vi "S4GUI.vi"(7 "Tab ObsEng":enum32{"Obs", "CCD modes", "Eng"}(tab)) -> ()   [LabVIEW 2018] (continued)
            w9668 = i16 1 items=["Cooler OFF", "Cooler ON"] ("Cooler ON/OFF")
          }
        }
        n4075 = Concatenate Strings("SET COOLER " ("User Event"), w9632, "CLICKED - CH4" ("User Event")) -> (w9636:string)
        n4076 = call-dynamic "Write User Event.vi"("error in (no error)"=w9633, "User Event"=w9636, "S4GUI in"=w9634) -> ("error out"=w9630:errorcluster, "S4GUI out"=w9631:refnum<class "S4GUI.lvclass">)  [unwired: 7 in]
        n4077 = call-dynamic "Read AcquisitionD.vi"("error in (no error)"=w9630, "S4ACS_GUI in"=w9631) -> ("error out"=w9640:errorcluster, "Acquisition.lvclass"=w9643:refnum<class "Acquisition.lvclass">, "S4ACS_GUI out"=w9644:refnum<class "S4GUI.lvclass">)  [unwired: 7 in]
        n4078 = call-dynamic "Read Channel.vi"("error in (no error)"=w9640, "Acquisition in"=w9643) -> ("error out"=w9649:errorcluster, "Channel.lvclass"=w9654:refnum<class "Channel.lvclass">, "Acquisition out"=w9657:refnum<class "Acquisition.lvclass">)  [unwired: 7 in]
        n4079 = call-dynamic "Read Interface.vi"("error in (no error)"=w9649, "Channel in"=w9654) -> ("error out"=w9648:errorcluster, "Interface.lvclass"=w9651:refnum<class "Interface.lvclass">, "Channel out"=w9653:refnum<class "Channel.lvclass">)  [unwired: 7 in]
        n4080 = call-dynamic "Write Cooler ON_OFF.vi"("error in (no error)"=w9648, "Cooler ON/OFF"=w9646, "Interface in"=w9651) -> ("error out"=w9647:errorcluster, "Interface out"=w9650:refnum<class "Interface.lvclass">)  [unwired: 7 in]
        n4081 = call-dynamic "Write Interface.vi"("error in (no error)"=w9647, "Interface.lvclass"=w9650, "Channel in"=w9653) -> ("error out"=w9639:errorcluster, "Channel out"=w9652:refnum<class "Channel.lvclass">)  [unwired: 7 in]
        n4082 = call-dynamic "Read State Machine.vi"("error in (no error)"=w9639, "Device in"=w9652) -> ("error out"=w9661:errorcluster, "State Machine.lvclass"=w9662:refnum<class "State Machine.lvclass">, "Device out"=w9658:refnum<class "Channel.lvclass">)  [unwired: 7 in]
        n4083 = call "Next State.vi"("error in (no error)"=w9661, "New_State"=u32 30, "State Machine in"=w9662) -> ("error out"=w9656:errorcluster, "State Machine out"=w9659:refnum<class "State Machine.lvclass">)  [unwired: 7 in]
        n4084 = call-dynamic "Write State Machine.vi"("error in (no error)"=w9656, "State Machine.lvclass"=w9659, "Device in"=w9658) -> ("error out"=w9655:errorcluster, "Device out"=w9645:refnum<class "Channel.lvclass">)  [unwired: 7 in]
        n4085 = call-dynamic "Write Channel.vi"("error in (no error)"=w9655, "Channel.lvclass"=w9645, "Acquisition in"=w9657) -> ("error out"=w9641:errorcluster, "Acquisition out"=w9642:refnum<class "Acquisition.lvclass">)  [unwired: 7 in]
        n4086 = call-dynamic "Write AcquisitionD.vi"("error in (no error)"=w9641, "Acquisition.lvclass"=w9642, "S4ACS_GUI in"=w9644) -> ("error out"=w9663:errorcluster, "S4ACS_GUI out"=w9664:refnum<class "S4GUI.lvclass">)  [unwired: 7 in]
      }
      event "Set Temp 1": Value Change {
        n4087 = event-data() -> ("NewVal"=w9669:bool)  [unwired: 1 in]
        n4088 = case shown="True" w9669 {
          tunnel: w9673 -> [w9675 w9702]
          tunnel: w9672 -> [w9674 w9701]
          tunnel: [w9674 w9691] -> w9671
          tunnel: [w9675 w9692] -> w9670
          frame False {
          }
          frame True {
            # "Carrega a maior temperatura\nentre target atual e o target do controle."
            # "Carrega o valor da temperatura target de acordo com a conf CCD"
            n4089 = call-dynamic "Read AcquisitionA.vi"("error in (no error)"=w9701, "S4ACS_GUI in"=w9702) -> ("error out"=w9705:errorcluster, "Acquisition.lvclass"=w9704:refnum<class "Acquisition.lvclass">, "S4ACS_GUI out"=w9711:refnum<class "S4GUI.lvclass">)  [unwired: 7 in]
            n4090 = call-dynamic "Read Channel.vi"("error in (no error)"=w9705, "Acquisition in"=w9704) -> ("error out"=w9721:errorcluster, "Channel.lvclass"=w9720:refnum<class "Channel.lvclass">, "Acquisition out"=w9708:refnum<class "Acquisition.lvclass">)  [unwired: 7 in]
            n4091 = call-dynamic "ValidateConfig.vi"("error in (no error)"=w9721, "Channel in"=w9720) -> ("error out"=w9727:errorcluster, "Channel out"=w9726:refnum<class "Channel.lvclass">)  [unwired: 7 in, 1 out]
            n4092 = call-dynamic "Read Interface.vi"("error in (no error)"=w9727, "Channel in"=w9726) -> ("error out"=w9723:errorcluster, "Interface.lvclass"=w9722:refnum<class "Interface.lvclass">, "Channel out"=w9716:refnum<class "Channel.lvclass">)  [unwired: 7 in]
            n4093 = call-dynamic "Read Temperature.vi"("error in (no error)"=w9723, "Interface in"=w9722) -> ("error out"=w9724:errorcluster, "Temperature"=w9729:i8, "Interface out"=w9725:refnum<class "Interface.lvclass">)  [unwired: 7 in]
            n4094 = Greater?(x=w9729, y="Target Temp 1") -> (0:w9728:bool)
            n4095 = Select(t=w9729, s=w9728, f="Target Temp 1") -> (s? t:f=w9695:i8)
            n4096 = call-dynamic "Write Temperature.vi"("error in (no error)"=w9724, "Temperature"=w9695, "Interface in"=w9725) -> ("error out"=w9718:errorcluster, "Interface out"=w9715:refnum<class "Interface.lvclass">)  [unwired: 7 in]
            n4097 = call-dynamic "Write Interface.vi"("error in (no error)"=w9718, "Interface.lvclass"=w9715, "Channel in"=w9716) -> ("error out"=w9719:errorcluster, "Channel out"=w9717:refnum<class "Channel.lvclass">)  [unwired: 7 in]
            n4098 = call-dynamic "Read State Machine.vi"("error in (no error)"=w9719, "Device in"=w9717) -> ("error out"=w9677:errorcluster, "State Machine.lvclass"=w9684:refnum<class "State Machine.lvclass">, "Device out"=w9707:refnum<class "Channel.lvclass">)  [unwired: 7 in]
            n4099 = call-dynamic "Read ref StatesQueue.vi"("error in (no error)"=w9677, "State Machine in"=w9684) -> ("error out"=w9687:errorcluster, "ref StatesQueue"=w9681:refnum<queue>, "State Machine out"=w9683:refnum<class "State Machine.lvclass">)  [unwired: 7 in]
            n4100 = Number To Decimal String(number="Target Temp 1") -> (decimal integer string=w9694:string)  [unwired: 1 in]
            n4101 = Flush Queue(queue=w9681, error in (no error)=w9687) -> (queue out=w9680:refnum<queue>, error out=w9689:errorcluster)  [unwired: 1 out]
            n4102 = Enqueue Element(queue=w9680, element=u32 35 ("State"), error in (no error)=w9689) -> (queue out=w9679:refnum<queue>, error out=w9690:errorcluster)  [unwired: 1 in, 1 out]
            n4103 = Enqueue Element(queue=w9679, element=u32 37 ("State"), error in (no error)=w9690) -> (queue out=w9678:refnum<queue>, error out=w9688:errorcluster)  [unwired: 1 in, 1 out]
            n4104 = call-dynamic "Write ref StatesQueue.vi"("error in (no error)"=w9688, "ref StatesQueue"=w9678, "State Machine in"=w9683) -> ("error out"=w9676:errorcluster, "State Machine out"=w9682:refnum<class "State Machine.lvclass">)  [unwired: 7 in]
            n4105 = call "Next State.vi"("error in (no error)"=w9676, "New_State"=u32 0, "State Machine in"=w9682) -> ("error out"=w9709:errorcluster, "State Machine out"=w9706:refnum<class "State Machine.lvclass">)  [unwired: 7 in]
            n4106 = call-dynamic "Write State Machine.vi"("error in (no error)"=w9709, "State Machine.lvclass"=w9706, "Device in"=w9707) -> ("error out"=w9713:errorcluster, "Device out"=w9714:refnum<class "Channel.lvclass">)  [unwired: 7 in]
            n4107 = call-dynamic "Write Channel.vi"("error in (no error)"=w9713, "Channel.lvclass"=w9714, "Acquisition in"=w9708) -> ("error out"=w9712:errorcluster, "Acquisition out"=w9710:refnum<class "Acquisition.lvclass">)  [unwired: 7 in]
            n4108 = call-dynamic "Write AcquisitionA.vi"("error in (no error)"=w9712, "Acquisition.lvclass"=w9710, "S4ACS_GUI in"=w9711) -> ("error out"=w9696:errorcluster, "S4ACS_GUI out"=w9697:refnum<class "S4GUI.lvclass">)  [unwired: 7 in]
            n4109 = Concatenate Strings("SET TEMP [" ("User Event"), w9694, "] CLICKED - CH1" ("User Event")) -> (w9700:string)
            n4110 = call-dynamic "Write User Event.vi"("error in (no error)"=w9696, "User Event"=w9700, "S4GUI in"=w9697) -> ("error out"=w9691:errorcluster, "S4GUI out"=w9692:refnum<class "S4GUI.lvclass">)  [unwired: 7 in]
          }
        }
      }
      event "Set Temp 2": Value Change {
        n4111 = event-data() -> ("NewVal"=w9730:bool)  [unwired: 1 in]
        n4112 = case shown="True" w9730 {
          tunnel: w9734 -> [w9736 w9762]
          tunnel: w9733 -> [w9735 w9761]
          tunnel: [w9735 w9754] -> w9732
          tunnel: [w9736 w9756] -> w9731
          frame False {
          }
          frame True {
            # "Carrega a maior temperatura\nentre target atual e o target do controle."
            # "Carrega o valor da temperatura target de acordo com a conf CCD"
            n4113 = call "Read AcquisitionB.vi"("error in (no error)"=w9761, "S4ACS_GUI in"=w9762) -> ("error out"=w9789:errorcluster, "Acquisition.lvclass"=w9790:refnum<class "Acquisition.lvclass">, "S4ACS_GUI out"=w9783:refnum<class "S4GUI.lvclass">)  [unwired: 7 in]
            n4114 = call-dynamic "Read Channel.vi"("error in (no error)"=w9789, "Acquisition in"=w9790) -> ("error out"=w9773:errorcluster, "Channel.lvclass"=w9774:refnum<class "Channel.lvclass">, "Acquisition out"=w9786:refnum<class "Acquisition.lvclass">)  [unwired: 7 in]
            n4115 = call-dynamic "ValidateConfig.vi"("error in (no error)"=w9773, "Channel in"=w9774) -> ("error out"=w9767:errorcluster, "Channel out"=w9768:refnum<class "Channel.lvclass">)  [unwired: 7 in, 1 out]
            n4116 = call-dynamic "Read Interface.vi"("error in (no error)"=w9767, "Channel in"=w9768) -> ("error out"=w9771:errorcluster, "Interface.lvclass"=w9772:refnum<class "Interface.lvclass">, "Channel out"=w9778:refnum<class "Channel.lvclass">)  [unwired: 7 in]
            n4117 = call-dynamic "Read Temperature.vi"("error in (no error)"=w9771, "Interface in"=w9772) -> ("error out"=w9770:errorcluster, "Temperature"=w9765:i8, "Interface out"=w9769:refnum<class "Interface.lvclass">)  [unwired: 7 in]
            n4118 = Greater?(x=w9765, y="Target Temp 2") -> (0:w9766:bool)
            n4119 = Select(t=w9765, s=w9766, f="Target Temp 2") -> (s? t:f=w9764:i32)
            n4120 = call-dynamic "Write Temperature.vi"("error in (no error)"=w9770, "Temperature"=w9764, "Interface in"=w9769) -> ("error out"=w9776:errorcluster, "Interface out"=w9779:refnum<class "Interface.lvclass">)  [unwired: 7 in]
            n4121 = call-dynamic "Write Interface.vi"("error in (no error)"=w9776, "Interface.lvclass"=w9779, "Channel in"=w9778) -> ("error out"=w9775:errorcluster, "Channel out"=w9777:refnum<class "Channel.lvclass">)  [unwired: 7 in]
            n4122 = call-dynamic "Read State Machine.vi"("error in (no error)"=w9775, "Device in"=w9777) -> ("error out"=w9737:errorcluster, "State Machine.lvclass"=w9740:refnum<class "State Machine.lvclass">, "Device out"=w9787:refnum<class "Channel.lvclass">)  [unwired: 7 in]
            n4123 = call-dynamic "Read ref StatesQueue.vi"("error in (no error)"=w9737, "State Machine in"=w9740) -> ("error out"=w9748:errorcluster, "ref StatesQueue"=w9743:refnum<queue>, "State Machine out"=w9741:refnum<class "State Machine.lvclass">)  [unwired: 7 in]
            n4124 = Flush Queue(queue=w9743, error in (no error)=w9748) -> (queue out=w9742:refnum<queue>, error out=w9750:errorcluster)  [unwired: 1 out]
            n4125 = Enqueue Element(queue=w9742, element=u32 35 ("State"), error in (no error)=w9750) -> (queue out=w9745:refnum<queue>, error out=w9751:errorcluster)  [unwired: 1 in, 1 out]
            n4126 = Enqueue Element(queue=w9745, element=u32 37 ("State"), error in (no error)=w9751) -> (queue out=w9744:refnum<queue>, error out=w9749:errorcluster)  [unwired: 1 in, 1 out]
            n4127 = call-dynamic "Write ref StatesQueue.vi"("error in (no error)"=w9749, "ref StatesQueue"=w9744, "State Machine in"=w9741) -> ("error out"=w9738:errorcluster, "State Machine out"=w9739:refnum<class "State Machine.lvclass">)  [unwired: 7 in]
            n4128 = call "Next State.vi"("error in (no error)"=w9738, "New_State"=u32 0, "State Machine in"=w9739) -> ("error out"=w9785:errorcluster, "State Machine out"=w9788:refnum<class "State Machine.lvclass">)  [unwired: 7 in]
            n4129 = call-dynamic "Write State Machine.vi"("error in (no error)"=w9785, "State Machine.lvclass"=w9788, "Device in"=w9787) -> ("error out"=w9781:errorcluster, "Device out"=w9780:refnum<class "Channel.lvclass">)  [unwired: 7 in]
            n4130 = Number To Decimal String(number="Target Temp 2") -> (decimal integer string=w9752:string)  [unwired: 1 in]
            n4131 = call-dynamic "Write Channel.vi"("error in (no error)"=w9781, "Channel.lvclass"=w9780, "Acquisition in"=w9786) -> ("error out"=w9782:errorcluster, "Acquisition out"=w9784:refnum<class "Acquisition.lvclass">)  [unwired: 7 in]
            n4132 = call "Write AcquisitionB.vi"("error in (no error)"=w9782, "Acquisition.lvclass"=w9784, "S4ACS_GUI in"=w9783) -> ("error out"=w9755:errorcluster, "S4ACS_GUI out"=w9757:refnum<class "S4GUI.lvclass">)  [unwired: 7 in]
            n4133 = Concatenate Strings("SET TEMP [" ("User Event"), w9752, "] CLICKED - CH2" ("User Event")) -> (w9760:string)
            n4134 = call-dynamic "Write User Event.vi"("error in (no error)"=w9755, "User Event"=w9760, "S4GUI in"=w9757) -> ("error out"=w9754:errorcluster, "S4GUI out"=w9756:refnum<class "S4GUI.lvclass">)  [unwired: 7 in]
          }
        }
      }
      event "Set Temp 3": Value Change {
        n4135 = event-data() -> ("NewVal"=w9791:bool)  [unwired: 1 in]
        n4136 = case shown="True" w9791 {
          tunnel: w9795 -> [w9797 w9823]
          tunnel: w9794 -> [w9796 w9822]
          tunnel: [w9796 w9814] -> w9793
          tunnel: [w9797 w9816] -> w9792
          frame False {
          }
          frame True {
            # "Carrega a maior temperatura\nentre target atual e o target do controle."
            # "Carrega o valor da temperatura target de acordo com a conf CCD"
            n4137 = call-dynamic "Read AcquisitionC.vi"("error in (no error)"=w9822, "S4ACS_GUI in"=w9823) -> ("error out"=w9825:errorcluster, "Acquisition.lvclass"=w9824:refnum<class "Acquisition.lvclass">, "S4ACS_GUI out"=w9832:refnum<class "S4GUI.lvclass">)  [unwired: 7 in]
            n4138 = call-dynamic "Read Channel.vi"("error in (no error)"=w9825, "Acquisition in"=w9824) -> ("error out"=w9842:errorcluster, "Channel.lvclass"=w9841:refnum<class "Channel.lvclass">, "Acquisition out"=w9829:refnum<class "Acquisition.lvclass">)  [unwired: 7 in]
            n4139 = call-dynamic "ValidateConfig.vi"("error in (no error)"=w9842, "Channel in"=w9841) -> ("error out"=w9848:errorcluster, "Channel out"=w9847:refnum<class "Channel.lvclass">)  [unwired: 7 in, 1 out]
            n4140 = call-dynamic "Read Interface.vi"("error in (no error)"=w9848, "Channel in"=w9847) -> ("error out"=w9844:errorcluster, "Interface.lvclass"=w9843:refnum<class "Interface.lvclass">, "Channel out"=w9837:refnum<class "Channel.lvclass">)  [unwired: 7 in]
            n4141 = call-dynamic "Read Temperature.vi"("error in (no error)"=w9844, "Interface in"=w9843) -> ("error out"=w9845:errorcluster, "Temperature"=w9850:i8, "Interface out"=w9846:refnum<class "Interface.lvclass">)  [unwired: 7 in]
            n4142 = Greater?(x=w9850, y="Target Temp 3") -> (0:w9849:bool)
            n4143 = Select(t=w9850, s=w9849, f="Target Temp 3") -> (s? t:f=w9851:i32)
            n4144 = call-dynamic "Write Temperature.vi"("error in (no error)"=w9845, "Temperature"=w9851, "Interface in"=w9846) -> ("error out"=w9839:errorcluster, "Interface out"=w9836:refnum<class "Interface.lvclass">)  [unwired: 7 in]
            n4145 = call-dynamic "Write Interface.vi"("error in (no error)"=w9839, "Interface.lvclass"=w9836, "Channel in"=w9837) -> ("error out"=w9840:errorcluster, "Channel out"=w9838:refnum<class "Channel.lvclass">)  [unwired: 7 in]
            n4146 = call-dynamic "Read State Machine.vi"("error in (no error)"=w9840, "Device in"=w9838) -> ("error out"=w9799:errorcluster, "State Machine.lvclass"=w9801:refnum<class "State Machine.lvclass">, "Device out"=w9828:refnum<class "Channel.lvclass">)  [unwired: 7 in]
            n4147 = call-dynamic "Read ref StatesQueue.vi"("error in (no error)"=w9799, "State Machine in"=w9801) -> ("error out"=w9807:errorcluster, "ref StatesQueue"=w9810:refnum<queue>, "State Machine out"=w9812:refnum<class "State Machine.lvclass">)  [unwired: 7 in]
            n4148 = Flush Queue(queue=w9810, error in (no error)=w9807) -> (queue out=w9811:refnum<queue>, error out=w9805:errorcluster)  [unwired: 1 out]
            n4149 = Enqueue Element(queue=w9811, element=u32 35 ("State"), error in (no error)=w9805) -> (queue out=w9808:refnum<queue>, error out=w9804:errorcluster)  [unwired: 1 in, 1 out]
            n4150 = Enqueue Element(queue=w9808, element=u32 37 ("State"), error in (no error)=w9804) -> (queue out=w9809:refnum<queue>, error out=w9806:errorcluster)  [unwired: 1 in, 1 out]
            n4151 = call-dynamic "Write ref StatesQueue.vi"("error in (no error)"=w9806, "ref StatesQueue"=w9809, "State Machine in"=w9812) -> ("error out"=w9798:errorcluster, "State Machine out"=w9800:refnum<class "State Machine.lvclass">)  [unwired: 7 in]
            n4152 = call "Next State.vi"("error in (no error)"=w9798, "New_State"=u32 0, "State Machine in"=w9800) -> ("error out"=w9830:errorcluster, "State Machine out"=w9827:refnum<class "State Machine.lvclass">)  [unwired: 7 in]
            n4153 = call-dynamic "Write State Machine.vi"("error in (no error)"=w9830, "State Machine.lvclass"=w9827, "Device in"=w9828) -> ("error out"=w9834:errorcluster, "Device out"=w9835:refnum<class "Channel.lvclass">)  [unwired: 7 in]
            n4154 = call-dynamic "Write Channel.vi"("error in (no error)"=w9834, "Channel.lvclass"=w9835, "Acquisition in"=w9829) -> ("error out"=w9833:errorcluster, "Acquisition out"=w9831:refnum<class "Acquisition.lvclass">)  [unwired: 7 in]
            n4155 = Number To Decimal String(number="Target Temp 3") -> (decimal integer string=w9818:string)  [unwired: 1 in]
            n4156 = call-dynamic "Write AcquisitionC.vi"("error in (no error)"=w9833, "Acquisition.lvclass"=w9831, "S4ACS_GUI in"=w9832) -> ("error out"=w9815:errorcluster, "S4ACS_GUI out"=w9817:refnum<class "S4GUI.lvclass">)  [unwired: 7 in]
            n4157 = Concatenate Strings("SET TEMP [" ("User Event"), w9818, "] CLICKED - CH3" ("User Event")) -> (w9821:string)
            n4158 = call-dynamic "Write User Event.vi"("error in (no error)"=w9815, "User Event"=w9821, "S4GUI in"=w9817) -> ("error out"=w9814:errorcluster, "S4GUI out"=w9816:refnum<class "S4GUI.lvclass">)  [unwired: 7 in]
          }
        }
      }
      event "Set Temp 4": Value Change {
        n4159 = event-data() -> ("NewVal"=w9852:bool)  [unwired: 1 in]
        n4160 = case shown="True" w9852 {
          tunnel: w9856 -> [w9858 w9900]
          tunnel: w9855 -> [w9857 w9899]
          tunnel: [w9857 w9874] -> w9854
          tunnel: [w9858 w9875] -> w9853
          frame False {
          }
          frame True {
            # "Carrega a maior temperatura\nentre target atual e o target do controle."
            # "Carrega o valor da temperatura target de acordo com a conf CCD"
            n4161 = call-dynamic "Read AcquisitionD.vi"("error in (no error)"=w9899, "S4ACS_GUI in"=w9900) -> ("error out"=w9911:errorcluster, "Acquisition.lvclass"=w9912:refnum<class "Acquisition.lvclass">, "S4ACS_GUI out"=w9904:refnum<class "S4GUI.lvclass">)  [unwired: 7 in]
            n4162 = call-dynamic "Read Channel.vi"("error in (no error)"=w9911, "Acquisition in"=w9912) -> ("error out"=w9892:errorcluster, "Channel.lvclass"=w9893:refnum<class "Channel.lvclass">, "Acquisition out"=w9907:refnum<class "Acquisition.lvclass">)  [unwired: 7 in]
            n4163 = call-dynamic "ValidateConfig.vi"("error in (no error)"=w9892, "Channel in"=w9893) -> ("error out"=w9886:errorcluster, "Channel out"=w9887:refnum<class "Channel.lvclass">)  [unwired: 7 in, 1 out]
            n4164 = call-dynamic "Read Interface.vi"("error in (no error)"=w9886, "Channel in"=w9887) -> ("error out"=w9890:errorcluster, "Interface.lvclass"=w9891:refnum<class "Interface.lvclass">, "Channel out"=w9897:refnum<class "Channel.lvclass">)  [unwired: 7 in]
            n4165 = call-dynamic "Read Temperature.vi"("error in (no error)"=w9890, "Interface in"=w9891) -> ("error out"=w9889:errorcluster, "Temperature"=w9884:i8, "Interface out"=w9888:refnum<class "Interface.lvclass">)  [unwired: 7 in]
            n4166 = Greater?(x=w9884, y="Target Temp 4") -> (0:w9885:bool)
            n4167 = Select(t=w9884, s=w9885, f="Target Temp 4") -> (s? t:f=w9883:i32)
            n4168 = call-dynamic "Write Temperature.vi"("error in (no error)"=w9889, "Temperature"=w9883, "Interface in"=w9888) -> ("error out"=w9895:errorcluster, "Interface out"=w9898:refnum<class "Interface.lvclass">)  [unwired: 7 in]
            n4169 = call-dynamic "Write Interface.vi"("error in (no error)"=w9895, "Interface.lvclass"=w9898, "Channel in"=w9897) -> ("error out"=w9894:errorcluster, "Channel out"=w9896:refnum<class "Channel.lvclass">)  [unwired: 7 in]
            n4170 = call-dynamic "Read State Machine.vi"("error in (no error)"=w9894, "Device in"=w9896) -> ("error out"=w9860:errorcluster, "State Machine.lvclass"=w9862:refnum<class "State Machine.lvclass">, "Device out"=w9908:refnum<class "Channel.lvclass">)  [unwired: 7 in]
            n4171 = call-dynamic "Read ref StatesQueue.vi"("error in (no error)"=w9860, "State Machine in"=w9862) -> ("error out"=w9870:errorcluster, "ref StatesQueue"=w9867:refnum<queue>, "State Machine out"=w9865:refnum<class "State Machine.lvclass">)  [unwired: 7 in]
            n4172 = Flush Queue(queue=w9867, error in (no error)=w9870) -> (queue out=w9866:refnum<queue>, error out=w9872:errorcluster)  [unwired: 1 out]
            n4173 = Enqueue Element(queue=w9866, element=u32 35 ("State"), error in (no error)=w9872) -> (queue out=w9869:refnum<queue>, error out=w9873:errorcluster)  [unwired: 1 in, 1 out]
            n4174 = Enqueue Element(queue=w9869, element=u32 37 ("State"), error in (no error)=w9873) -> (queue out=w9868:refnum<queue>, error out=w9871:errorcluster)  [unwired: 1 in, 1 out]
            n4175 = call-dynamic "Write ref StatesQueue.vi"("error in (no error)"=w9871, "ref StatesQueue"=w9868, "State Machine in"=w9865) -> ("error out"=w9859:errorcluster, "State Machine out"=w9861:refnum<class "State Machine.lvclass">)  [unwired: 7 in]
            n4176 = call "Next State.vi"("error in (no error)"=w9859, "New_State"=u32 0, "State Machine in"=w9861) -> ("error out"=w9906:errorcluster, "State Machine out"=w9909:refnum<class "State Machine.lvclass">)  [unwired: 7 in]
            n4177 = call-dynamic "Write State Machine.vi"("error in (no error)"=w9906, "State Machine.lvclass"=w9909, "Device in"=w9908) -> ("error out"=w9902:errorcluster, "Device out"=w9901:refnum<class "Channel.lvclass">)  [unwired: 7 in]
            n4178 = Number To Decimal String(number="Target Temp 4") -> (decimal integer string=w9882:string)  [unwired: 1 in]
            n4179 = call-dynamic "Write Channel.vi"("error in (no error)"=w9902, "Channel.lvclass"=w9901, "Acquisition in"=w9907) -> ("error out"=w9903:errorcluster, "Acquisition out"=w9905:refnum<class "Acquisition.lvclass">)  [unwired: 7 in]
            n4180 = call-dynamic "Write AcquisitionD.vi"("error in (no error)"=w9903, "Acquisition.lvclass"=w9905, "S4ACS_GUI in"=w9904) -> ("error out"=w9876:errorcluster, "S4ACS_GUI out"=w9877:refnum<class "S4GUI.lvclass">)  [unwired: 7 in]
            n4181 = Concatenate Strings("SET TEMP [" ("User Event"), w9882, "] CLICKED - CH4" ("User Event")) -> (w9881:string)
            n4182 = call-dynamic "Write User Event.vi"("error in (no error)"=w9876, "User Event"=w9881, "S4GUI in"=w9877) -> ("error out"=w9874:errorcluster, "S4GUI out"=w9875:refnum<class "S4GUI.lvclass">)  [unwired: 7 in]
          }
        }
      }
      event "Avança Estado": Value Change {
        n4183 = event-data() -> ()  [unwired: 1 in, 4 out]
        n4184 = call-dynamic "Read Sync Box.lvclass.vi"("error in (no error)"=w9921, "SPARC4_AC in"=w9922) -> ("error out"=w9934:errorcluster, "Sync Box.lvclass"=w9935:refnum<class "Sync Box.lvclass">, "SPARC4_AC out"=w9926:refnum<class "S4GUI.lvclass">)  [unwired: 7 in]
        n4185 = call-dynamic "Read Trigger.lvclass.vi"("error in (no error)"=w9934, "Sync Box in"=w9935) -> ("error out"=w9932:errorcluster, "Trigger.lvclass"=w9933:refnum<class "Trigger.lvclass">, "Sync Box out"=w9929:refnum<class "Sync Box.lvclass">)  [unwired: 7 in]
        n4186 = call-dynamic "Read State Machine.vi"("error in (no error)"=w9932, "Device in"=w9933) -> ("error out"=w9918:errorcluster, "State Machine.lvclass"=w9919:refnum<class "State Machine.lvclass">, "Device out"=w9930:refnum<class "Trigger.lvclass">)  [unwired: 7 in]
        n4187 = call-dynamic "Read State.vi"("error in (no error)"=w9918, "State Machine in"=w9919) -> ("error out"=w9914:errorcluster, "State"=w9917:i32, "State Machine out"=w9915:refnum<class "State Machine.lvclass">)  [unwired: 7 in]
        n4188 = Increment(x=w9917) -> (x+1=w9916:i32)
        n4189 = call "Next State.vi"("error in (no error)"=w9914, "New_State"=w9916, "State Machine in"=w9915) -> ("error out"=w9928:errorcluster, "State Machine out"=w9931:refnum<class "State Machine.lvclass">)  [unwired: 7 in]
        n4190 = call-dynamic "Write State Machine.vi"("error in (no error)"=w9928, "State Machine.lvclass"=w9931, "Device in"=w9930) -> ("error out"=w9924:errorcluster, "Device out"=w9923:refnum<class "Trigger.lvclass">)  [unwired: 7 in]
        n4191 = call-dynamic "Write Trigger.lvclass.vi"("error in (no error)"=w9924, "Trigger.lvclass"=w9923, "Sync Box in"=w9929) -> ("error out"=w9925:errorcluster, "Sync Box out"=w9927:refnum<class "Sync Box.lvclass">)  [unwired: 7 in]
        n4192 = call-dynamic "Write Sync Box.lvclass.vi"("error in (no error)"=w9925, "Sync Box.lvclass"=w9927, "SPARC4_AC in"=w9926) -> ("error out"=w9920:errorcluster, "SPARC4_AC out"=w9913:refnum<class "S4GUI.lvclass">)  [unwired: 7 in]
      }
      event "DelayA": Value Change {
        n4193 = event-data() -> ("NewVal"=w9937:string)  [unwired: 1 in, 3 out]
        n4194 = call-dynamic "Read Sync Box.lvclass.vi"("error in (no error)"=w9941, "SPARC4_AC in"=w9942) -> ("error out"=w9949:errorcluster, "Sync Box.lvclass"=w9950:refnum<class "Sync Box.lvclass">, "SPARC4_AC out"=w9946:refnum<class "S4GUI.lvclass">)  [unwired: 7 in]
        n4195 = call-dynamic "Read Trigger.lvclass.vi"("error in (no error)"=w9949, "Sync Box in"=w9950) -> ("error out"=w9938:errorcluster, "Trigger.lvclass"=w9939:refnum<class "Trigger.lvclass">, "Sync Box out"=w9948:refnum<class "Sync Box.lvclass">)  [unwired: 7 in]
        n4196 = call-dynamic "Write DelayA.vi"("error in (no error)"=w9938, "DelayA"=w9937, "Trigger in"=w9939) -> ("error out"=w9944:errorcluster, "Trigger out"=w9943:refnum<class "Trigger.lvclass">)  [unwired: 7 in]
        n4197 = call-dynamic "Write Trigger.lvclass.vi"("error in (no error)"=w9944, "Trigger.lvclass"=w9943, "Sync Box in"=w9948) -> ("error out"=w9945:errorcluster, "Sync Box out"=w9947:refnum<class "Sync Box.lvclass">)  [unwired: 7 in]
        n4198 = call-dynamic "Write Sync Box.lvclass.vi"("error in (no error)"=w9945, "Sync Box.lvclass"=w9947, "SPARC4_AC in"=w9946) -> ("error out"=w9940:errorcluster, "SPARC4_AC out"=w9936:refnum<class "S4GUI.lvclass">)  [unwired: 7 in]
      }
      event "DelayB": Value Change {
        n4199 = event-data() -> ("NewVal"=w9952:string)  [unwired: 1 in, 3 out]
        n4200 = call-dynamic "Read Sync Box.lvclass.vi"("error in (no error)"=w9956, "SPARC4_AC in"=w9957) -> ("error out"=w9964:errorcluster, "Sync Box.lvclass"=w9965:refnum<class "Sync Box.lvclass">, "SPARC4_AC out"=w9961:refnum<class "S4GUI.lvclass">)  [unwired: 7 in]
        n4201 = call-dynamic "Read Trigger.lvclass.vi"("error in (no error)"=w9964, "Sync Box in"=w9965) -> ("error out"=w9953:errorcluster, "Trigger.lvclass"=w9954:refnum<class "Trigger.lvclass">, "Sync Box out"=w9963:refnum<class "Sync Box.lvclass">)  [unwired: 7 in]
        n4202 = call-dynamic "Write DelayB.vi"("error in (no error)"=w9953, "DelayB"=w9952, "Trigger in"=w9954) -> ("error out"=w9959:errorcluster, "Trigger out"=w9958:refnum<class "Trigger.lvclass">)  [unwired: 7 in]
        n4203 = call-dynamic "Write Trigger.lvclass.vi"("error in (no error)"=w9959, "Trigger.lvclass"=w9958, "Sync Box in"=w9963) -> ("error out"=w9960:errorcluster, "Sync Box out"=w9962:refnum<class "Sync Box.lvclass">)  [unwired: 7 in]
        n4204 = call-dynamic "Write Sync Box.lvclass.vi"("error in (no error)"=w9960, "Sync Box.lvclass"=w9962, "SPARC4_AC in"=w9961) -> ("error out"=w9955:errorcluster, "SPARC4_AC out"=w9951:refnum<class "S4GUI.lvclass">)  [unwired: 7 in]
      }
      event "DelayC": Value Change {
        n4205 = event-data() -> ("NewVal"=w9967:string)  [unwired: 1 in, 3 out]
        n4206 = call-dynamic "Read Sync Box.lvclass.vi"("error in (no error)"=w9971, "SPARC4_AC in"=w9972) -> ("error out"=w9979:errorcluster, "Sync Box.lvclass"=w9980:refnum<class "Sync Box.lvclass">, "SPARC4_AC out"=w9976:refnum<class "S4GUI.lvclass">)  [unwired: 7 in]
        n4207 = call-dynamic "Read Trigger.lvclass.vi"("error in (no error)"=w9979, "Sync Box in"=w9980) -> ("error out"=w9968:errorcluster, "Trigger.lvclass"=w9969:refnum<class "Trigger.lvclass">, "Sync Box out"=w9978:refnum<class "Sync Box.lvclass">)  [unwired: 7 in]
        n4208 = call-dynamic "Write DelayC.vi"("error in (no error)"=w9968, "DelayC"=w9967, "Trigger in"=w9969) -> ("error out"=w9974:errorcluster, "Trigger out"=w9973:refnum<class "Trigger.lvclass">)  [unwired: 7 in]
        n4209 = call-dynamic "Write Trigger.lvclass.vi"("error in (no error)"=w9974, "Trigger.lvclass"=w9973, "Sync Box in"=w9978) -> ("error out"=w9975:errorcluster, "Sync Box out"=w9977:refnum<class "Sync Box.lvclass">)  [unwired: 7 in]
        n4210 = call-dynamic "Write Sync Box.lvclass.vi"("error in (no error)"=w9975, "Sync Box.lvclass"=w9977, "SPARC4_AC in"=w9976) -> ("error out"=w9970:errorcluster, "SPARC4_AC out"=w9966:refnum<class "S4GUI.lvclass">)  [unwired: 7 in]
      }
      event "DelayD": Value Change {
        n4211 = event-data() -> ("NewVal"=w9982:string)  [unwired: 1 in, 3 out]
        n4212 = call-dynamic "Read Sync Box.lvclass.vi"("error in (no error)"=w9986, "SPARC4_AC in"=w9987) -> ("error out"=w9994:errorcluster, "Sync Box.lvclass"=w9995:refnum<class "Sync Box.lvclass">, "SPARC4_AC out"=w9991:refnum<class "S4GUI.lvclass">)  [unwired: 7 in]
        n4213 = call-dynamic "Read Trigger.lvclass.vi"("error in (no error)"=w9994, "Sync Box in"=w9995) -> ("error out"=w9983:errorcluster, "Trigger.lvclass"=w9984:refnum<class "Trigger.lvclass">, "Sync Box out"=w9993:refnum<class "Sync Box.lvclass">)  [unwired: 7 in]
        n4214 = call-dynamic "Write DelayD.vi"("error in (no error)"=w9983, "DelayD"=w9982, "Trigger in"=w9984) -> ("error out"=w9989:errorcluster, "Trigger out"=w9988:refnum<class "Trigger.lvclass">)  [unwired: 7 in]
        n4215 = call-dynamic "Write Trigger.lvclass.vi"("error in (no error)"=w9989, "Trigger.lvclass"=w9988, "Sync Box in"=w9993) -> ("error out"=w9990:errorcluster, "Sync Box out"=w9992:refnum<class "Sync Box.lvclass">)  [unwired: 7 in]
        n4216 = call-dynamic "Write Sync Box.lvclass.vi"("error in (no error)"=w9990, "Sync Box.lvclass"=w9992, "SPARC4_AC in"=w9991) -> ("error out"=w9985:errorcluster, "SPARC4_AC out"=w9981:refnum<class "S4GUI.lvclass">)  [unwired: 7 in]
      }
      event "WidthA": Value Change {
        n4217 = event-data() -> ("NewVal"=w9997:string)  [unwired: 1 in, 3 out]
        n4218 = call-dynamic "Read Sync Box.lvclass.vi"("error in (no error)"=w10001, "SPARC4_AC in"=w10002) -> ("error out"=w10009:errorcluster, "Sync Box.lvclass"=w10010:refnum<class "Sync Box.lvclass">, "SPARC4_AC out"=w10006:refnum<class "S4GUI.lvclass">)  [unwired: 7 in]
        n4219 = call-dynamic "Read Trigger.lvclass.vi"("error in (no error)"=w10009, "Sync Box in"=w10010) -> ("error out"=w9998:errorcluster, "Trigger.lvclass"=w9999:refnum<class "Trigger.lvclass">, "Sync Box out"=w10008:refnum<class "Sync Box.lvclass">)  [unwired: 7 in]
        n4220 = call-dynamic "Write WidthA.vi"("error in (no error)"=w9998, "WidthA"=w9997, "Trigger in"=w9999) -> ("error out"=w10004:errorcluster, "Trigger out"=w10003:refnum<class "Trigger.lvclass">)  [unwired: 7 in]
        n4221 = call-dynamic "Write Trigger.lvclass.vi"("error in (no error)"=w10004, "Trigger.lvclass"=w10003, "Sync Box in"=w10008) -> ("error out"=w10005:errorcluster, "Sync Box out"=w10007:refnum<class "Sync Box.lvclass">)  [unwired: 7 in]
        n4222 = call-dynamic "Write Sync Box.lvclass.vi"("error in (no error)"=w10005, "Sync Box.lvclass"=w10007, "SPARC4_AC in"=w10006) -> ("error out"=w10000:errorcluster, "SPARC4_AC out"=w9996:refnum<class "S4GUI.lvclass">)  [unwired: 7 in]
      }
      event "WidthB": Value Change {
        n4223 = event-data() -> ("NewVal"=w10012:string)  [unwired: 1 in, 3 out]
        n4224 = call-dynamic "Read Sync Box.lvclass.vi"("error in (no error)"=w10016, "SPARC4_AC in"=w10017) -> ("error out"=w10024:errorcluster, "Sync Box.lvclass"=w10025:refnum<class "Sync Box.lvclass">, "SPARC4_AC out"=w10021:refnum<class "S4GUI.lvclass">)  [unwired: 7 in]
        n4225 = call-dynamic "Read Trigger.lvclass.vi"("error in (no error)"=w10024, "Sync Box in"=w10025) -> ("error out"=w10013:errorcluster, "Trigger.lvclass"=w10014:refnum<class "Trigger.lvclass">, "Sync Box out"=w10023:refnum<class "Sync Box.lvclass">)  [unwired: 7 in]
        n4226 = call-dynamic "Write WidthB.vi"("error in (no error)"=w10013, "WidthB"=w10012, "Trigger in"=w10014) -> ("error out"=w10019:errorcluster, "Trigger out"=w10018:refnum<class "Trigger.lvclass">)  [unwired: 7 in]
        n4227 = call-dynamic "Write Trigger.lvclass.vi"("error in (no error)"=w10019, "Trigger.lvclass"=w10018, "Sync Box in"=w10023) -> ("error out"=w10020:errorcluster, "Sync Box out"=w10022:refnum<class "Sync Box.lvclass">)  [unwired: 7 in]
        n4228 = call-dynamic "Write Sync Box.lvclass.vi"("error in (no error)"=w10020, "Sync Box.lvclass"=w10022, "SPARC4_AC in"=w10021) -> ("error out"=w10015:errorcluster, "SPARC4_AC out"=w10011:refnum<class "S4GUI.lvclass">)  [unwired: 7 in]
      }
      event "WidthC": Value Change {
        n4229 = event-data() -> ("NewVal"=w10027:string)  [unwired: 1 in, 3 out]
        n4230 = call-dynamic "Read Sync Box.lvclass.vi"("error in (no error)"=w10031, "SPARC4_AC in"=w10032) -> ("error out"=w10039:errorcluster, "Sync Box.lvclass"=w10040:refnum<class "Sync Box.lvclass">, "SPARC4_AC out"=w10036:refnum<class "S4GUI.lvclass">)  [unwired: 7 in]
        n4231 = call-dynamic "Read Trigger.lvclass.vi"("error in (no error)"=w10039, "Sync Box in"=w10040) -> ("error out"=w10028:errorcluster, "Trigger.lvclass"=w10029:refnum<class "Trigger.lvclass">, "Sync Box out"=w10038:refnum<class "Sync Box.lvclass">)  [unwired: 7 in]
        n4232 = call-dynamic "Write WidthC.vi"("error in (no error)"=w10028, "WidthC"=w10027, "Trigger in"=w10029) -> ("error out"=w10034:errorcluster, "Trigger out"=w10033:refnum<class "Trigger.lvclass">)  [unwired: 7 in]
        n4233 = call-dynamic "Write Trigger.lvclass.vi"("error in (no error)"=w10034, "Trigger.lvclass"=w10033, "Sync Box in"=w10038) -> ("error out"=w10035:errorcluster, "Sync Box out"=w10037:refnum<class "Sync Box.lvclass">)  [unwired: 7 in]
        n4234 = call-dynamic "Write Sync Box.lvclass.vi"("error in (no error)"=w10035, "Sync Box.lvclass"=w10037, "SPARC4_AC in"=w10036) -> ("error out"=w10030:errorcluster, "SPARC4_AC out"=w10026:refnum<class "S4GUI.lvclass">)  [unwired: 7 in]
      }
      event "WidthD": Value Change {
        n4235 = event-data() -> ("NewVal"=w10042:string)  [unwired: 1 in, 3 out]
        n4236 = call-dynamic "Read Sync Box.lvclass.vi"("error in (no error)"=w10046, "SPARC4_AC in"=w10047) -> ("error out"=w10054:errorcluster, "Sync Box.lvclass"=w10055:refnum<class "Sync Box.lvclass">, "SPARC4_AC out"=w10051:refnum<class "S4GUI.lvclass">)  [unwired: 7 in]
        n4237 = call-dynamic "Read Trigger.lvclass.vi"("error in (no error)"=w10054, "Sync Box in"=w10055) -> ("error out"=w10043:errorcluster, "Trigger.lvclass"=w10044:refnum<class "Trigger.lvclass">, "Sync Box out"=w10053:refnum<class "Sync Box.lvclass">)  [unwired: 7 in]
        n4238 = call-dynamic "Write WidthD.vi"("error in (no error)"=w10043, "WidthD"=w10042, "Trigger in"=w10044) -> ("error out"=w10049:errorcluster, "Trigger out"=w10048:refnum<class "Trigger.lvclass">)  [unwired: 7 in]
        n4239 = call-dynamic "Write Trigger.lvclass.vi"("error in (no error)"=w10049, "Trigger.lvclass"=w10048, "Sync Box in"=w10053) -> ("error out"=w10050:errorcluster, "Sync Box out"=w10052:refnum<class "Sync Box.lvclass">)  [unwired: 7 in]
        n4240 = call-dynamic "Write Sync Box.lvclass.vi"("error in (no error)"=w10050, "Sync Box.lvclass"=w10052, "SPARC4_AC in"=w10051) -> ("error out"=w10045:errorcluster, "SPARC4_AC out"=w10041:refnum<class "S4GUI.lvclass">)  [unwired: 7 in]
      }
      event "WPROT_set": Value Change {
        # "Espera até 10 x 1s = 10s\npara condition de WPROT\n ir para READY"
        n4241 = event-data() -> ()  [unwired: 1 in, 4 out]
        n4242 = call "Read Instrument.lvclass.vi"("error in (no error)"=w10077, "S4ACS_GUI in"=w10078) -> ("error out"=w10075:errorcluster, "Instrument.lvclass"=w10076:refnum<class "Instrument.lvclass">, "S4ACS_GUI out"=w10064:refnum<class "S4GUI.lvclass">)  [unwired: 7 in]
        n4243 = call "Read WPROT.vi"("error in (no error)"=w10075, "Instrument in"=w10076) -> ("error out"=w10071:errorcluster, "Opt_Selector.lvclass"=w10074:refnum<class "Opt_Selector.lvclass">, "Instrument out"=w10067:refnum<class "Instrument.lvclass">)  [unwired: 7 in]
        n4244 = call-dynamic "Read State Machine.vi"("error in (no error)"=w10071, "Device in"=w10074) -> ("error out"=w10070:errorcluster, "State Machine.lvclass"=w10073:refnum<class "State Machine.lvclass">, "Device out"=w10069:refnum<class "Opt_Selector.lvclass">)  [unwired: 7 in]
        n4245 = call "Next State.vi"("error in (no error)"=w10070, "New_State"=1, "State Machine in"=w10073) -> ("error out"=w10058:errorcluster, "State Machine out"=w10060:refnum<class "State Machine.lvclass">)  [unwired: 7 in]
        n4246 = call-dynamic "Write Timer.vi"("error in (no error)"=w10058, "Timer"=u32 10, "State Machine in"=w10060) -> ("error out"=w10057:errorcluster, "State Machine out"=w10059:refnum<class "State Machine.lvclass">)  [unwired: 7 in]
        n4247 = call-dynamic "Write State Machine.vi"("error in (no error)"=w10057, "State Machine.lvclass"=w10059, "Device in"=w10069) -> ("error out"=w10066:errorcluster, "Device out"=w10068:refnum<class "Opt_Selector.lvclass">)  [unwired: 7 in]
        n4248 = call "Write WPROT.vi"("error in (no error)"=w10066, "Opt_Selector.lvclass"=w10068, "Instrument in"=w10067) -> ("error out"=w10063:errorcluster, "Instrument out"=w10065:refnum<class "Instrument.lvclass">)  [unwired: 7 in]
        n4249 = call "Write Instrument.lvclass.vi"("error in (no error)"=w10063, "Instrument.lvclass"=w10065, "S4ACS_GUI in"=w10064) -> ("error out"=w10062:errorcluster, "S4ACS_GUI out"=w10061:refnum<class "S4GUI.lvclass">)  [unwired: 7 in]
      }
      event "TARGET NAME WPROT": Value Change {
        n4250 = event-data() -> ()  [unwired: 1 in, 1 out]
        n4251 = call "Read Instrument.lvclass.vi"("error in (no error)"=w10106, "S4ACS_GUI in"=w10107) -> ("error out"=w10114:errorcluster, "Instrument.lvclass"=w10115:refnum<class "Instrument.lvclass">, "S4ACS_GUI out"=w10109:refnum<class "S4GUI.lvclass">)  [unwired: 7 in]
        n4252 = property on="TARGET NAME WPROT" class="Enum (strict)"() -> ("RingText.Text"=w10105:string)  [unwired: 2 in, 2 out]
        n4253 = Build Array(-1.0 ("element"), 0.0 ("element"), 22.5 ("element"), 45.0 ("element"), 67.5 ("element"), 90.0 ("element"), 112.5 ("element"), 135.0 ("element"), 157.5 ("element"), 180.0 ("element"), 202.5 ("element"), 225.0 ("element"), 247.5 ("element"), 270.0 ("element"), 292.5 ("element"), 315.0 ("element"), 337.5 ("element")) -> (w10097:dbl[])
        n4254 = call "Read WPROT.vi"("error in (no error)"=w10114, "Instrument in"=w10115) -> ("error out"=w10112:errorcluster, "Opt_Selector.lvclass"=w10113:refnum<class "Opt_Selector.lvclass">, "Instrument out"=w10111:refnum<class "Instrument.lvclass">)  [unwired: 7 in]
        n4255 = call "Write target name.vi"("error in (no error)"=w10112, "target name"=w10105, "Optics in"=w10113) -> ("error out"=w10093:errorcluster, "Optics out"=w10094:refnum<class "Opt_Selector.lvclass">)  [unwired: 7 in]
        n4256 = Index Array(array=w10097, index="TARGET NAME WPROT") -> (element=w10095:dbl)
        n4257 = call "Write target.vi"("error in (no error)"=w10093, "target"=w10095, "Optics in"=w10094) -> ("error out"=w10092:errorcluster, "Optics out"=w10091:refnum<class "Opt_Selector.lvclass">)  [unwired: 7 in]
        n4258 = call "Write WPROT.vi"("error in (no error)"=w10092, "Opt_Selector.lvclass"=w10091, "Instrument in"=w10111) -> ("error out"=w10108:errorcluster, "Instrument out"=w10110:refnum<class "Instrument.lvclass">)  [unwired: 7 in]
        n4259 = call "Write Instrument.lvclass.vi"("error in (no error)"=w10108, "Instrument.lvclass"=w10110, "S4ACS_GUI in"=w10109) -> ("error out"=w10104:errorcluster, "S4ACS_GUI out"=w10079:refnum<class "S4GUI.lvclass">)  [unwired: 7 in]
      }
      event "TARGET NAME WPSEL": Value Change {
        n4260 = event-data() -> ()  [unwired: 1 in, 1 out]
        n4261 = call "Read Instrument.lvclass.vi"("error in (no error)"=w10130, "S4ACS_GUI in"=w10131) -> ("error out"=w10138:errorcluster, "Instrument.lvclass"=w10139:refnum<class "Instrument.lvclass">, "S4ACS_GUI out"=w10133:refnum<class "S4GUI.lvclass">)  [unwired: 7 in]
        n4262 = property on="TARGET NAME WPSEL" class="Enum (strict)"() -> ("RingText.Text"=w10117:string)  [unwired: 2 in, 2 out]
        n4263 = Build Array(-1.0 ("element"), 80.0 ("element"), 0.0 ("element"), 160.0 ("element")) -> (w10124:dbl[])
        n4264 = call "Read WPSEL.vi"("error in (no error)"=w10138, "Instrument in"=w10139) -> ("error out"=w10136:errorcluster, "Opt_Selector.lvclass"=w10137:refnum<class "Opt_Selector.lvclass">, "Instrument out"=w10135:refnum<class "Instrument.lvclass">)  [unwired: 7 in]
        n4265 = call "Write target name.vi"("error in (no error)"=w10136, "target name"=w10117, "Optics in"=w10137) -> ("error out"=w10121:errorcluster, "Optics out"=w10122:refnum<class "Opt_Selector.lvclass">)  [unwired: 7 in]
        n4266 = Index Array(array=w10124, index="TARGET NAME WPSEL") -> (element=w10123:dbl)
        n4267 = call "Write target.vi"("error in (no error)"=w10121, "target"=w10123, "Optics in"=w10122) -> ("error out"=w10120:errorcluster, "Optics out"=w10119:refnum<class "Opt_Selector.lvclass">)  [unwired: 7 in]
        n4268 = call "Write WPSEL.vi"("error in (no error)"=w10120, "Opt_Selector.lvclass"=w10119, "Instrument in"=w10135) -> ("error out"=w10132:errorcluster, "Instrument out"=w10134:refnum<class "Instrument.lvclass">)  [unwired: 7 in]
        n4269 = call "Write Instrument.lvclass.vi"("error in (no error)"=w10132, "Instrument.lvclass"=w10134, "S4ACS_GUI in"=w10133) -> ("error out"=w10129:errorcluster, "S4ACS_GUI out"=w10116:refnum<class "S4GUI.lvclass">)  [unwired: 7 in]
      }
      event "Lambda Selector": Value Change {
        n4270 = event-data() -> ("NewVal"=w10141:u16)  [unwired: 1 in, 1 out]
        n4271 = call "Read Instrument.lvclass.vi"("error in (no error)"=w10172, "S4ACS_GUI in"=w10173) -> ("error out"=w10174:errorcluster, "Instrument.lvclass"=w10149:refnum<class "Instrument.lvclass">, "S4ACS_GUI out"=w10146:refnum<class "S4GUI.lvclass">)  [unwired: 7 in]
        n4272 = Build Array(80.0 ("element"), 0.0 ("element"), 160.0 ("element")) -> (w10167:dbl[])
        n4273 = property on="Lambda Selector" class="Ring (strict)"() -> ("RingText.Text"=w10147:string)  [unwired: 2 in, 2 out]
        n4274 = call "Read WPSEL.vi"("error in (no error)"=w10174, "Instrument in"=w10149) -> ("error out"=w10156:errorcluster, "Opt_Selector.lvclass"=w10155:refnum<class "Opt_Selector.lvclass">, "Instrument out"=w10148:refnum<class "Instrument.lvclass">)  [unwired: 7 in]
        n4275 = Index Array(array=w10167, index=w10141) -> (element=w10166:dbl)
        n4276 = call "Write target.vi"("error in (no error)"=w10156, "target"=w10166, "Optics in"=w10155) -> ("error out"=w10153:errorcluster, "Optics out"=w10154:refnum<class "Opt_Selector.lvclass">)  [unwired: 7 in]
        n4277 = case shown="\"Lambda/4\"" w10147 {
          selector: w10147 -> [w10177 _ _]
          tunnel: [w10177 "ON" "ON"] -> w10158
          tunnel: [0.0 ("element") 30.0 ("element") 30.0 ("element")] -> w10157
          tunnel: [w10177 "L/2" "L/4"] -> w10150
          frame "OFF", Default {
            n4278 = property on="Calibrator Selector" class="Ring (strict)"("DisabledEnum"=T12."Disabled and Grayed Out" ("Disabled")) -> ()  [unwired: 2 in, 2 out]
          }
          frame "Lambda/2" {
            n4279 = property on="Calibrator Selector" class="Ring (strict)"("DisabledEnum"=T12."Enabled" ("Disabled")) -> ()  [unwired: 2 in, 2 out]
          }
          frame "Lambda/4" {
            n4280 = property on="Calibrator Selector" class="Ring (strict)"("DisabledEnum"=T12."Enabled" ("Disabled")) -> ()  [unwired: 2 in, 2 out]
          }
        }
        n4281 = call "Write target name.vi"("error in (no error)"=w10153, "target name"=w10150, "Optics in"=w10154) -> ("error out"=w10152:errorcluster, "Optics out"=w10151:refnum<class "Opt_Selector.lvclass">)  [unwired: 7 in]
        n4282 = call "Write WPSEL.vi"("error in (no error)"=w10152, "Opt_Selector.lvclass"=w10151, "Instrument in"=w10148) -> ("error out"=w10143:errorcluster, "Instrument out"=w10142:refnum<class "Instrument.lvclass">)  [unwired: 7 in]
        n4283 = call "Read ASEL.vi"("error in (no error)"=w10143, "Instrument in"=w10142) -> ("error out"=w10163:errorcluster, "Opt_Selector.lvclass"=w10161:refnum<class "Opt_Selector.lvclass">, "Instrument out"=w10145:refnum<class "Instrument.lvclass">)  [unwired: 7 in]
        n4284 = call "Write target name.vi"("error in (no error)"=w10163, "target name"=w10158, "Optics in"=w10161) -> ("error out"=w10164:errorcluster, "Optics out"=w10160:refnum<class "Opt_Selector.lvclass">)  [unwired: 7 in]
        n4285 = call "Write target.vi"("error in (no error)"=w10164, "target"=w10157, "Optics in"=w10160) -> ("error out"=w10165:errorcluster, "Optics out"=w10159:refnum<class "Opt_Selector.lvclass">)  [unwired: 7 in]
        n4286 = call "Write ASEL.vi"("error in (no error)"=w10165, "Opt_Selector.lvclass"=w10159, "Instrument in"=w10145) -> ("error out"=w10162:errorcluster, "Instrument out"=w10144:refnum<class "Instrument.lvclass">)  [unwired: 7 in]
        n4287 = call "Write Instrument.lvclass.vi"("error in (no error)"=w10162, "Instrument.lvclass"=w10144, "S4ACS_GUI in"=w10146) -> ("error out"=w10171:errorcluster, "S4ACS_GUI out"=w10140:refnum<class "S4GUI.lvclass">)  [unwired: 7 in]
      }
      event "Calibrator Selector": Value Change {
        n4288 = event-data() -> ()  [unwired: 1 in, 6 out]
        n4289 = call "Read Instrument.lvclass.vi"("error in (no error)"=w10206, "S4ACS_GUI in"=w10207) -> ("error out"=w10210:errorcluster, "Instrument.lvclass"=w10211:refnum<class "Instrument.lvclass">, "S4ACS_GUI out"=w10208:refnum<class "S4GUI.lvclass">)  [unwired: 7 in]
        n4290 = Build Array(0.0 ("element"), 72.0 ("element"), 144.0 ("element"), 216.0 ("element"), 288.0 ("element")) -> (w10201:dbl[])
        n4291 = call "Read CALW.vi"("error in (no error)"=w10210, "Instrument in"=w10211) -> ("error out"=w10199:errorcluster, "Opt_Selector.lvclass"=w10198:refnum<class "Opt_Selector.lvclass">, "Instrument out"=w10209:refnum<class "Instrument.lvclass">)  [unwired: 7 in]
        n4292 = Index Array(array=w10201, index="Calibrator Selector") -> (element=w10200:dbl)
        n4293 = call "Write target.vi"("error in (no error)"=w10199, "target"=w10200, "Optics in"=w10198) -> ("error out"=w10196:errorcluster, "Optics out"=w10197:refnum<class "Opt_Selector.lvclass">)  [unwired: 7 in]
        n4294 = property on="Calibrator Selector" class="Ring (strict)"() -> ("RingText.Text"=w10192:string)  [unwired: 2 in, 2 out]
        n4295 = case shown="\"POLARIZER\"" w10192 {
          selector: w10192 -> [_ w10213 w10214 w10215 w10216]
          tunnel: ["OFF" w10213 w10214 w10215 w10216] -> w10193
          frame "OFF", Default {
          }
          frame "POLARIZER" {
          }
          frame "DEPOLARIZER" {
          }
          frame "PINHOLE" {
          }
          frame "SHUTTER" {
          }
        }
        n4296 = call "Write target name.vi"("error in (no error)"=w10196, "target name"=w10193, "Optics in"=w10197) -> ("error out"=w10195:errorcluster, "Optics out"=w10194:refnum<class "Opt_Selector.lvclass">)  [unwired: 7 in]
        n4297 = call "Write CALW.vi"("error in (no error)"=w10195, "Opt_Selector.lvclass"=w10194, "Instrument in"=w10209) -> ("error out"=w10189:errorcluster, "Instrument out"=w10190:refnum<class "Instrument.lvclass">)  [unwired: 7 in]
        n4298 = call "Write Instrument.lvclass.vi"("error in (no error)"=w10189, "Instrument.lvclass"=w10190, "S4ACS_GUI in"=w10208) -> ("error out"=w10205:errorcluster, "S4ACS_GUI out"=w10188:refnum<class "S4GUI.lvclass">)  [unwired: 7 in]
      }
      event "TARGET NAME CALW": Value Change {
        # "aqui também"
        # "OV20230825: Valores da sequência original"
        n4299 = event-data() -> ()  [unwired: 1 in, 6 out]
        n4300 = call "Read Instrument.lvclass.vi"("error in (no error)"=w10233, "S4ACS_GUI in"=w10234) -> ("error out"=w10241:errorcluster, "Instrument.lvclass"=w10242:refnum<class "Instrument.lvclass">, "S4ACS_GUI out"=w10236:refnum<class "S4GUI.lvclass">)  [unwired: 7 in]
        n4301 = property on="TARGET NAME CALW" class="Enum (strict)"() -> ("RingText.Text"=w10217:string)  [unwired: 2 in, 2 out]
        n4302 = Build Array(-1.0 ("element"), 0.0 ("element"), 72.0 ("element"), 144.0 ("element"), 216.0 ("element"), 288.0 ("element")) -> (w10227:dbl[])
        n4303 = call "Read CALW.vi"("error in (no error)"=w10241, "Instrument in"=w10242) -> ("error out"=w10239:errorcluster, "Opt_Selector.lvclass"=w10240:refnum<class "Opt_Selector.lvclass">, "Instrument out"=w10238:refnum<class "Instrument.lvclass">)  [unwired: 7 in]
        n4304 = call "Write target name.vi"("error in (no error)"=w10239, "target name"=w10217, "Optics in"=w10240) -> ("error out"=w10224:errorcluster, "Optics out"=w10225:refnum<class "Opt_Selector.lvclass">)  [unwired: 7 in]
        n4305 = Index Array(array=w10227, index="TARGET NAME CALW") -> (element=w10226:dbl)
        n4306 = call "Write target.vi"("error in (no error)"=w10224, "target"=w10226, "Optics in"=w10225) -> ("error out"=w10223:errorcluster, "Optics out"=w10222:refnum<class "Opt_Selector.lvclass">)  [unwired: 7 in]
        n4307 = call "Write CALW.vi"("error in (no error)"=w10223, "Opt_Selector.lvclass"=w10222, "Instrument in"=w10238) -> ("error out"=w10235:errorcluster, "Instrument out"=w10237:refnum<class "Instrument.lvclass">)  [unwired: 7 in]
        n4308 = call "Write Instrument.lvclass.vi"("error in (no error)"=w10235, "Instrument.lvclass"=w10237, "S4ACS_GUI in"=w10236) -> ("error out"=w10232:errorcluster, "S4ACS_GUI out"=w10218:refnum<class "S4GUI.lvclass">)  [unwired: 7 in]
      }
      event "TARGET NAME ASEL": Value Change {
        n4309 = event-data() -> ()  [unwired: 1 in, 6 out]
        n4310 = call "Read Instrument.lvclass.vi"("error in (no error)"=w10256, "S4ACS_GUI in"=w10257) -> ("error out"=w10264:errorcluster, "Instrument.lvclass"=w10265:refnum<class "Instrument.lvclass">, "S4ACS_GUI out"=w10259:refnum<class "S4GUI.lvclass">)  [unwired: 7 in]
        n4311 = Build Array(-1.0 ("element"), 0.0 ("element"), 30.0 ("element")) -> (w10251:dbl[])
        n4312 = call "Read ASEL.vi"("error in (no error)"=w10264, "Instrument in"=w10265) -> ("error out"=w10262:errorcluster, "Opt_Selector.lvclass"=w10263:refnum<class "Opt_Selector.lvclass">, "Instrument out"=w10261:refnum<class "Instrument.lvclass">)  [unwired: 7 in]
